vi "do_section_analysis.vi"(8 "Error In":errorcluster) -> (0 "Error Out":errorcluster)   [LabVIEW 2019]
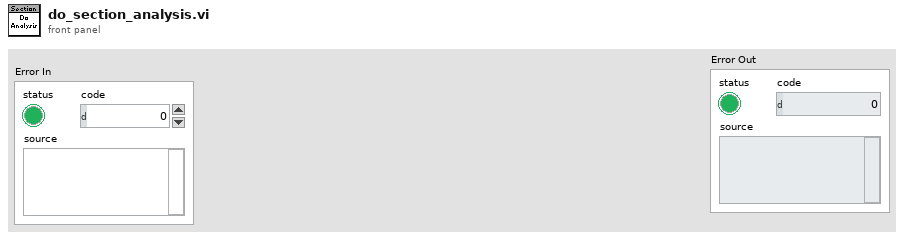
[diagram p1: front panel]
types:
  T1 = typedef "section_parameters_cluster_typedef.ctl" = cluster{"Section":string, "Method":T2, "Edge Mode":T3, "ROI Size":T4, "Manual Sequence":T5, "Grid Constant":i32, "Min Grain Size":dbl, "Comments":string, "File Path":path}
  T2 = typedef "sections_method_enum_typedef.ctl" = enum16{"Edge Detection", "Grid Only", "Manual Selection", "Existing Edges"}
  T3 = typedef "sections_edge_mode_enum_typedef.ctl" = enum16{"Grid for Large Grains Only", "Grid", "No Grid"}
  T4 = typedef "sections_roi_size_enum_typedef.ctl" = enum16{"0x0", "1x1", "2x2", "3x3", "4x4", "5x5", "6x6"}
  T5 = typedef "xi_angles_enum_typedef.ctl" = enum16{"0", "45"}
  T6 = typedef "parameters_cluster_typedef.ctl" = cluster{"m1":dbl, "m2":dbl, "m3":dbl, "c":dbl, "D":dbl, "Beta":dbl, "center x":dbl, "center y":dbl}
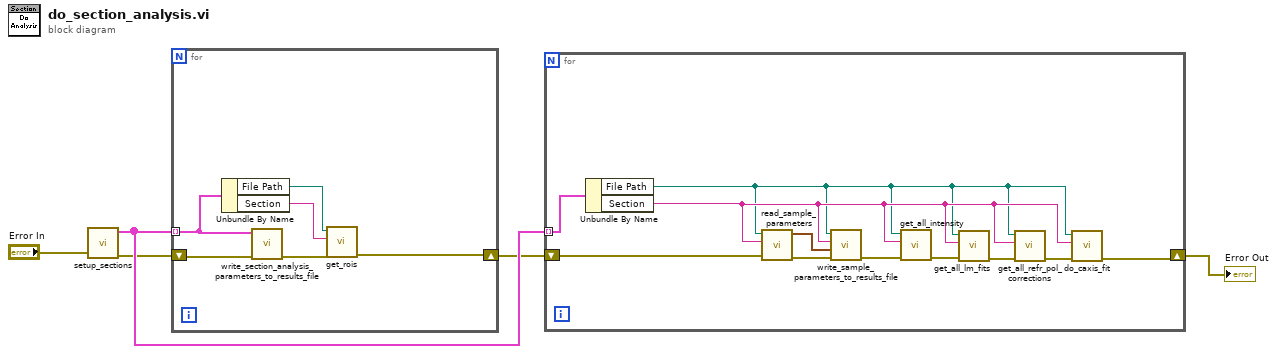
[diagram p0: block diagram]
diagram:
  n1 = call "setup_sections.vi"("Error In"="Error In") -> ("Error Out"=w2:errorcluster, "Parameters Array"=w3:T1[])  [unwired: 9 in]
  n2 = for {
    tunnel: [w7] -> _ mode=indexing
    tunnel: w3 -> [w7] mode=indexing
    shift-right: [w6] -> w1
    shift-left: w2 -> [w8]
    n3 = Unbundle By Name(w7) -> ("File Path"=w10:path, "Section"=w9:string)
    n4 = call "write_section_analysis_parameters_to_results_file.vi"("Error In"=w8, "Section Parameters"=w7) -> ("Error Out"=w11:errorcluster)  [unwired: 9 in]
    n5 = call "get_rois.vi"("Error In"=w11, "Sample"=w9, "File Path"=w10) -> ("Error Out"=w6:errorcluster)  [unwired: 8 in]
  }
  n6 = for {
    shift-right: [w15] -> w4
    shift-left: w1 -> [w16]
    tunnel: w3 -> [w18] mode=indexing
    n7 = Unbundle By Name(w18) -> ("File Path"=w12:path, "Section"=w13:string)
    n8 = call "read_sample_parameters.vi"("Error In"=w16, "Sample"=w13, "File Path"=w12) -> ("Error Out"=w22:errorcluster, "Parameters"=w20:T6)  [unwired: 6 in, 1 out]
    n9 = call "write_sample_parameters_to_results_file.vi"("Error In"=w22, "Parameters"=w20, "Sample"=w13, "File Path"=w12) -> ("Error Out"=w21:errorcluster)  [unwired: 7 in]
    n10 = call "get_all_intensity.vi"("Error In"=w21, "Sample"=w13, "File Path"=w12) -> ("Error Out"=w19:errorcluster)  [unwired: 8 in]
    n11 = call "get_all_lm_fits.vi"("Error In"=w19, "Sample"=w13, "File Path"=w12) -> ("Error Out"=w17:errorcluster)  [unwired: 8 in]
    n12 = call "get_all_refr_pol_corrections.vi"("Error In"=w17, "Sample"=w13, "File Path"=w12) -> ("Error Out"=w14:errorcluster)  [unwired: 8 in]
    n13 = call "do_caxis_fit.vi"("Error In"=w14, "Sample"=w13, "File Path"=w12) -> ("Error Out"=w15:errorcluster)  [unwired: 8 in]
  }
  "Error Out" <- w4
